vi "NextState.vi"(0 "object in":refnum<class "KickTactic.lvclass">, 2 "Robot in":refnum<class "Robot.lvclass">, 4 "GameRef":refnum<data-value>, 5 "error in (no error)":errorcluster) -> (14 "object out":refnum<class "KickTactic.lvclass">, 19 "error out":errorcluster)   [LabVIEW 2023, in "KickTactic.lvclass"]
uses:
  KickTactic.lvclass
  C:/Users/ebert/Documents/codes/SSL/repo/SSL_AI/NewSTP/NewTactics/Tactic_v2_class/Tactic_v2.lvclass
  Robot_class/Robot.lvclass
  Game_class/Game.lvclass
  KickTactic_states_class/KickTactic_states.ctl
  KickTactic.lvclass/KickTactic.ctl
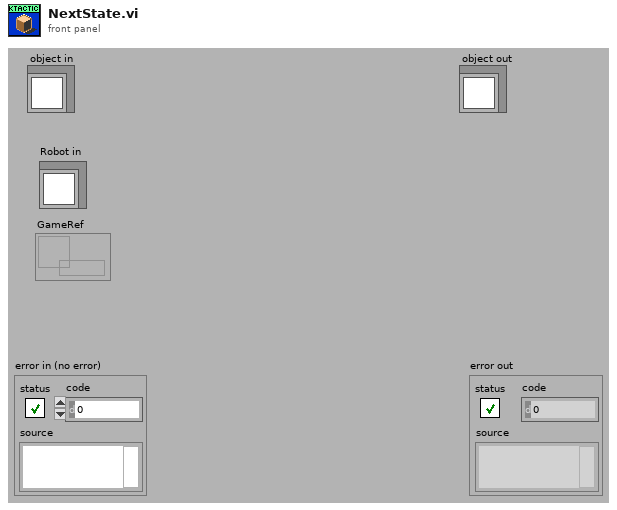
[diagram p1: front panel]
types:
  T1 = typedef "KickTactic.lvclass/KickTactic_states.ctl" = enum16{"GoToTangentPoint", "Circulate", "Align", "Kick"}
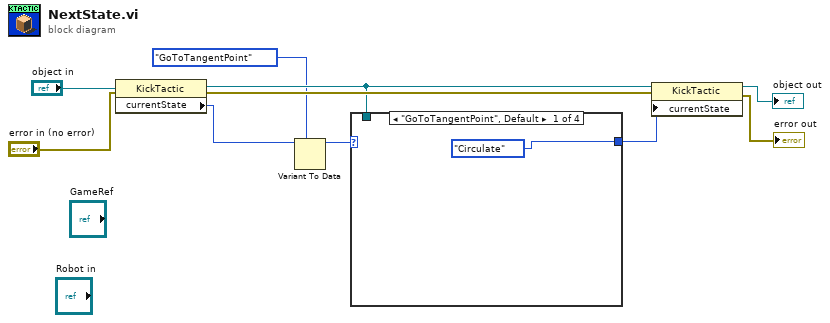
[diagram p0: block diagram]
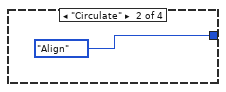
[diagram p2: hidden frame]
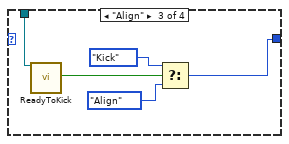
[diagram p3: hidden frame]
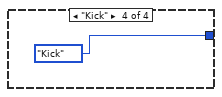
[diagram p4: hidden frame]
diagram:
  n1 = property class="KickTactic"(reference="object in", error in="error in (no error)") -> (reference out=w4:refnum<class "KickTactic.lvclass">, error out=w6:errorcluster, "currentState"=w3:u8)
  n2 = Variant To Data(type=KickTactic_states."GoToTangentPoint" ("Enum"), Variant=w3) -> (data=w1:T1)  [unwired: 1 in, 1 out]
  n3 = case shown="\"GoToTangentPoint\", Default" w1 {
    tunnel: [KickTactic_states."Circulate" ("Enum") KickTactic_states."Align" ("Enum") w13 KickTactic_states."Kick" ("Enum")] -> w9
    tunnel: w4 -> [_ _ w17 _]
    frame "GoToTangentPoint", Default {
    }
    frame "Circulate" {
    }
    frame "Align" {
      n4 = call-dynamic "ReadyToKick.vi"("object in"=w17) -> ("ready"=w16:bool)  [unwired: 16 in, 2 out]
      n5 = Select(t=KickTactic_states."Kick" ("Enum"), s=w16, f=KickTactic_states."Align" ("Enum")) -> (s? t:f=w13:T1)
    }
    frame "Kick" {
    }
  }
  n6 = property class="KickTactic"(reference=w4, error in=w6, "currentState"=w9) -> (reference out=→"object out":refnum<class "KickTactic.lvclass">, error out=→"error out":errorcluster)
